vi "Introspection Core.vi"(8 "error in (no error)":errorcluster, 11 "CS++DSMonitor in":refnum<class "CS++DSMonitor.lvclass">) -> (0 "error out":errorcluster, 2 "CS++Messages":refnum<class "Message.lvclass">[](array[class]), 3 "CS++DSMonitor out":refnum<class "CS++DSMonitor.lvclass">)   [LabVIEW 2016, in "CS++DSMonitor.lvlib" / "CS++DSMonitor.lvclass"]
doc: "This vi delivers a list with all messages this actor reacts to. \n\nNote that all inherited classes have to overwrite it."
uses:
  CS++DSMonitor.lvclass
  <vilib>/ActorFramework/Message/Message.lvclass
  CS++PVMonitor/CS++PVMonitor.lvclass
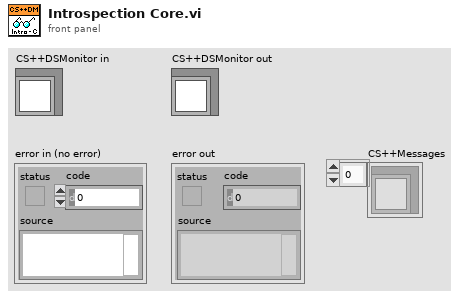
[diagram p1: front panel]
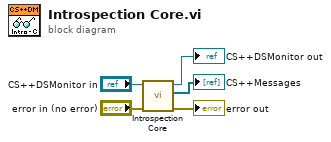
[diagram p0: block diagram]
diagram:
  n1 = call-parent "Introspection Core.vi"("error in (no error)"="error in (no error)", "CS++PVMonitor in"="CS++DSMonitor in") -> ("error out"=→"error out":errorcluster, "CS++Messages"=→"CS++Messages":refnum<class "Message.lvclass">[], "CS++PVMonitor out"=→"CS++DSMonitor out":refnum<class "CS++DSMonitor.lvclass">)  [unwired: 7 in]
